vi "Get-PAQ-tags.vi"(8 "error in (no error)":errorcluster, 11 "HISW in":refnum<class "HISW.lvclass">) -> (0 "error out":errorcluster, 2 "PAQ_TAGs":string[](array[string]), 3 "HISW out":refnum<class "HISW.lvclass">)   [LabVIEW 2014, in "HISW.lvclass"]
doc: "Read TAGs of Qtype : PAQ"
uses:
  HISW.lvclass
  FAMM/FAMM.lvclass
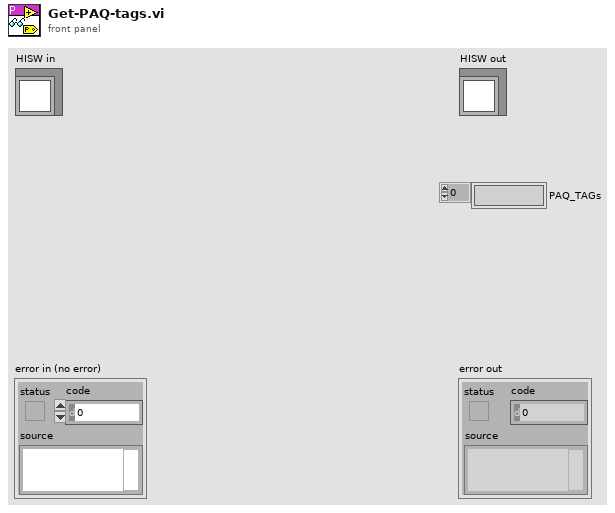
[diagram p1: front panel]
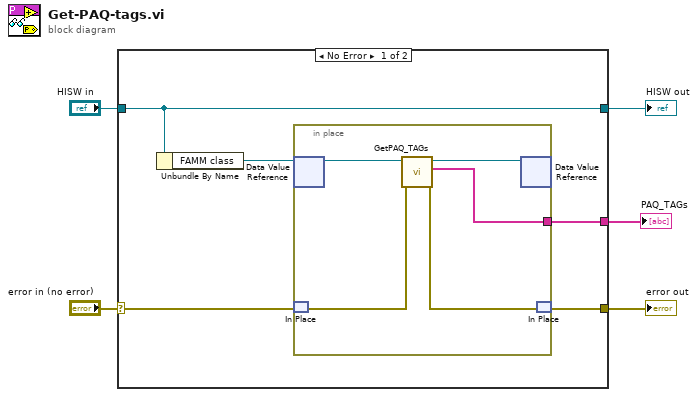
[diagram p0: block diagram]
diagram:
  n1 = case shown="No Error" "error in (no error)" {
    selector: "error in (no error)" -> [w8 w17]
    tunnel: [w7 w17] -> w4
    tunnel: [w10 w16] -> w2
    tunnel: "HISW in" -> [w10 w16]
    tunnel: [w6 _] -> w1
    frame No Error {
      n2 = Unbundle By Name(w10) -> ("FAMM class"=w9:refnum<data-value>)
      n3 = in-place {
        in-place-border: [w11] -> w6
        n4 = in-place-dvr #1(w9) -> (w15:refnum<class "FAMM.lvclass">)  [unwired: 1 out]
        n5 = in-place-match #2(w8) -> (w13:errorcluster)
        n6 = call "GetPAQ_TAGs.vi"("error in (no error)"=w13, "FAMM in"=w15) -> ("error out"=w12:errorcluster, "PAQ_TAGs"=w11:string[], "FAMM out"=w14:refnum<class "FAMM.lvclass">)  [unwired: 7 in]
        n7 = in-place-dvr #1(w14) -> ()  [unwired: 2 out]
        n8 = in-place-match #2(w12) -> (w7:errorcluster)
      }
    }
    frame Error {
    }
  }
  "error out" <- w4
  "HISW out" <- w2
  "PAQ_TAGs" <- w1
